vi "Temp ctrl age.vi"(8 "Gas conc":dbl, 9 "Flow rate":dbl, 10 "Tgas":dbl, 11 "Delta T":dbl) -> (2 "Gas MF":dbl)   [LabVIEW 2011]
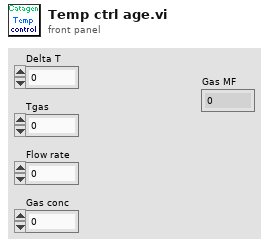
[diagram p1: front panel]
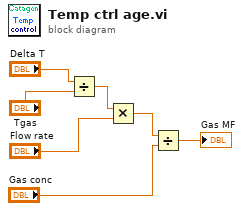
[diagram p0: block diagram]
diagram:
  n1 = Divide(x="Delta T", y="Tgas") -> (x/y=w5:dbl)
  n2 = Multiply(x=w5, y="Flow rate") -> (x*y=w3:dbl)
  n3 = Divide(x=w3, y="Gas conc") -> (x/y=→"Gas MF":dbl)
